vi "ControllerMain.vi"(0 "AllData":T1, 5 "PID gains":T5={"proportional gain (Kc)"=1.0, "integral time (Ti, min)"=0.01, "derivative time (Td, min)"=0.0} {"derivative time (Td, min)" format="%.3f"; "integral time (Ti, min)" format="%.3f"; "proportional gain (Kc)" format="%.3f"}, 7 "AdmittanceCoeffs":T4, 11 "error in (no error)":errorcluster) -> (4 "U1":dbl, 6 "Direction1":bool, 8 "U2":dbl, 10 "Direction 2":bool, 15 "error out":errorcluster)   [LabVIEW 2017, in "admittanceControllerLibrary.lvlib"]
doc: "The VI is the Admittance Controller Main API.\n\nInputs: All Data, PID Gains, Admittance Coeefficients.\n\nOutputs: Motor 1 demand and direction. Motor 2 demand and direction."
uses:
  admittanceControllerLibrary.lvlib
  Controls/AdmittanceGains.ctl
  TypeDefs/allData.ctl
  TypeDefs/dataOut.ctl
  TypeDefs/dataIn.ctl
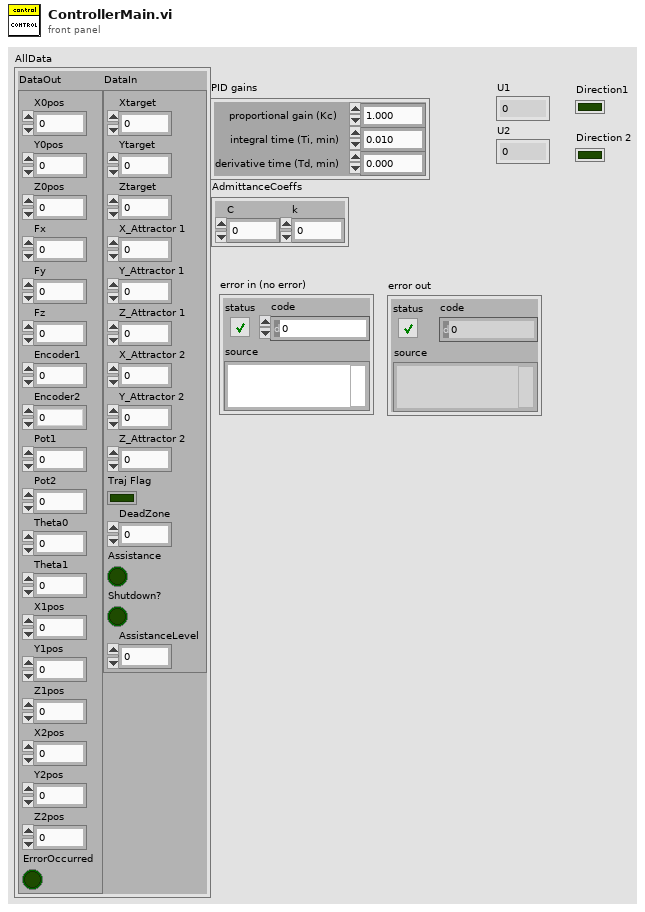
[diagram p1: front panel]
types:
  T1 = typedef "allData.ctl" = cluster{"DataOut":T2, "DataIn":T3}
  T2 = typedef "dataOut.ctl" = cluster{"X0pos":dbl, "Y0pos":dbl, "Z0pos":dbl, "Fx":dbl, "Fy":dbl, "Fz":dbl, "Encoder1":i32, "Encoder2":i32, "Pot1":dbl, "Pot2":dbl, "Theta0":dbl, "Theta1":dbl, "X1pos":dbl, "Y1pos":dbl, "Z1pos":dbl, "X2pos":dbl, "Y2pos":dbl, "Z2pos":dbl, "ErrorOccurred":bool}
  T3 = typedef "dataIn.ctl" = cluster{"Xtarget":dbl, "Ytarget":dbl, "Ztarget":dbl, "X_Attractor 1":dbl, "Y_Attractor 1":dbl, "Z_Attractor 1":dbl, "X_Attractor 2":dbl, "Y_Attractor 2":dbl, "Z_Attractor 2":dbl, "Traj Flag":bool, "DeadZone":dbl, "Assistance":bool, "Shutdown?":bool, "AssistanceLevel":dbl}
  T4 = typedef "admittanceControllerLibrary.lvlib/AdmittanceGains.ctl" = cluster{"C":dbl, "k":dbl}
  T5 = cluster{"proportional gain (Kc)":dbl, "integral time (Ti, min)":dbl, "derivative time (Td, min)":dbl}
  T6 = typedef "admittanceControllerLibrary.lvlib/ControlVariables.ctl" = cluster{"ControlFlag":bool, "Fx":dbl, "Fy":dbl, "Theta0":dbl, "Theta1":dbl, "CurrentX":dbl, "CurrentY":dbl, "TargetX":dbl, "TargetY":dbl, "DeadZone":dbl, "Assistance?":bool, "AssitanceLevel":dbl}
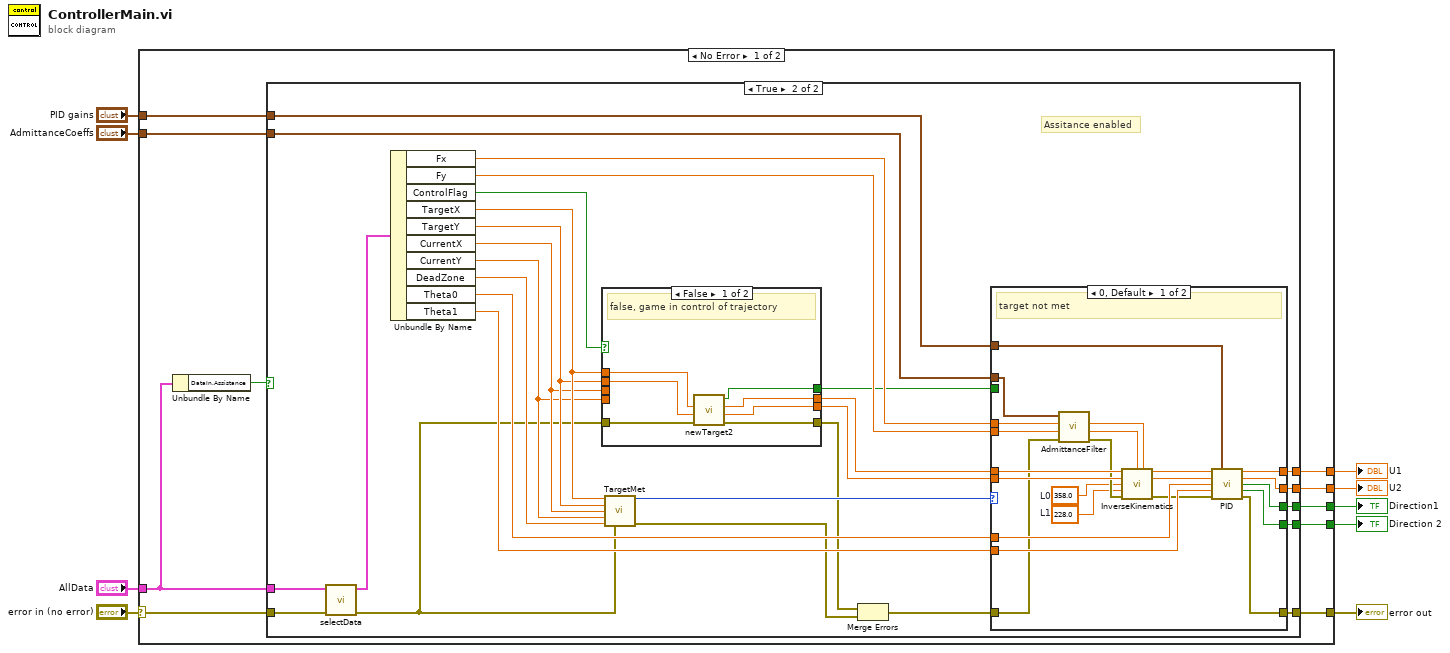
[diagram p0: block diagram]
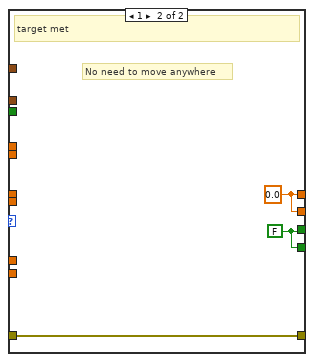
[diagram p3: hidden frame]
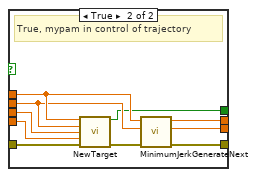
[diagram p4: hidden frame]
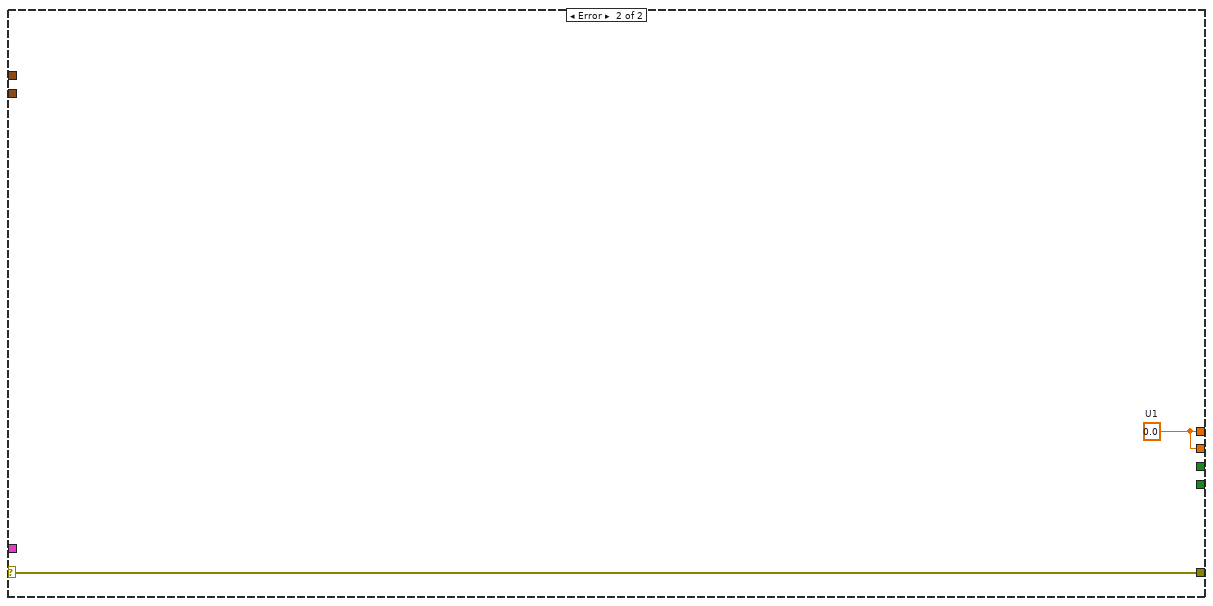
[diagram p5: hidden frame]
diagram:
  n1 = case shown="No Error" "error in (no error)" {
    selector: "error in (no error)" -> [w15 w92]
    tunnel: [w19 w91] -> w9
    tunnel: [w18 w91] -> w8
    tunnel: "PID gains" -> [w11 _]
    tunnel: "AdmittanceCoeffs" -> [w12 _]
    tunnel: [w17 _] -> w5
    tunnel: [w16 _] -> w4
    tunnel: [w14 w92] -> w2
    tunnel: "AllData" -> [w13 _]
    frame No Error {
      n2 = Unbundle By Name(w13) -> ("DataIn.Assistance"=w10:bool)
      n3 = case shown="True" w10 {
        tunnel: [_ w39] -> w19
        tunnel: [_ w38] -> w18
        tunnel: [_ w33] -> w17
        tunnel: [_ w32] -> w16
        tunnel: w15 -> [w20 w30]
        tunnel: [w20 w25] -> w14
        tunnel: w13 -> [_ w24]
        tunnel: w12 -> [_ w23]
        tunnel: w11 -> [_ w22]
        frame False {
          # "Assistance not enabled"
        }
        frame True {
          # "Assitance enabled"
          n4 = call "selectData.vi"("error in (no error)"=w30, "AllData"=w24) -> ("error out"=w27:errorcluster, 3:w31:T6)  [unwired: 8 in]
          n5 = Unbundle By Name(w31) -> ("Fx"=w36:dbl, "Fy"=w37:dbl, "ControlFlag"=w48:bool, "TargetX"=w47:dbl, "TargetY"=w46:dbl, "CurrentX"=w45:dbl, "CurrentY"=w44:dbl, "DeadZone"=w43:dbl, "Theta0"=w34:dbl, "Theta1"=w35:dbl)
          n6 = case shown="False" w48 {
            tunnel: w47 -> [w75 w88]
            tunnel: w46 -> [w74 w87]
            tunnel: w45 -> [_ w86]
            tunnel: w44 -> [_ w85]
            tunnel: [w77 w90] -> w41
            tunnel: [w78 w89] -> w40
            tunnel: w27 -> [w80 w84]
            tunnel: [w79 w82] -> w29
            tunnel: [w76 w81] -> w21
            frame False {
              # "false, game in control of trajectory"
              n7 = call "newTarget2.vi"("error in (no error)"=w80, "Target Y"=w74, "Target X"=w75) -> ("error out"=w79:errorcluster, "Target y"=w78:dbl, "Target x"=w77:dbl, "NewTarget"=w76:bool)  [unwired: 5 in]
            }
            frame True {
              # "True, mypam in control of trajectory"
              n8 = call "NewTarget.vi"("Target x"=w88, "Target y"=w87, "Current x"=w86, "Current y"=w85, "error in (no error)"=w84) -> ("NewTarget"=w81:bool, "error out"=w83:errorcluster)  [unwired: 9 in]
              n9 = call "MinimumJerkGenerateNext.vi"("error in (no error)"=w83, "Target y"=w87, "Target x"=w88) -> ("error out"=w82:errorcluster, "yt"=w89:dbl, "xt"=w90:dbl)  [unwired: 6 in]
            }
          }
          n10 = call "TargetMet.vi"("Target x (mm)"=w47, "Target y (mm)"=w46, "Current x (mm)"=w45, "Current y (mm)"=w44, "Dead Zone (mm)"=w43, "error in (no error)"=w27) -> ("out"=w42:i32, "error out"=w28:errorcluster)  [unwired: 8 in]
          n11 = Merge Errors(w29, w28) -> (w26:errorcluster)
          n12 = case shown="0, Default" w42 {
            tunnel: w41 -> [w61 _]
            tunnel: w40 -> [w60 _]
            tunnel: [w66 w73] -> w39
            tunnel: [w67 w73] -> w38
            tunnel: w36 -> [w63 _]
            tunnel: w37 -> [w62 _]
            tunnel: w34 -> [w69 _]
            tunnel: w35 -> [w68 _]
            tunnel: w22 -> [w70 _]
            tunnel: [w65 w72] -> w33
            tunnel: [w64 w72] -> w32
            tunnel: w26 -> [w56 w71]
            tunnel: [w58 w71] -> w25
            tunnel: w23 -> [w49 _]
            tunnel: w21 -> [_ _]
            frame 0, Default {
              w50 = 228.0  # L1
              w51 = 358.0  # L0
              # "target not met"
              n13 = call "AdmittanceFilter.vi"("error in (no error)"=w56, "Fy"=w62, "Fx"=w63, "AdmittanceCoeffs"=w49) -> ("error out"=w57:errorcluster, "Delta y"=w55:dbl, "Delta x"=w54:dbl)  [unwired: 5 in]
              n14 = call "InverseKinematics.vi"("Next X"=w61, "deltaY"=w55, "deltaX"=w54, "Next Y"=w60, "L0"=w51, "L1"=w50, "error in (no error)"=w57) -> ("destheta0"=w53:dbl, "destheta1"=w52:dbl, "error out"=w59:errorcluster)  [unwired: 6 in]
              n15 = call "PID.vi"("Des theta0"=w53, "PID gains"=w70, "Des theta1"=w52, "current theta0"=w69, "current theta1"=w68, "error in (no error)"=w59) -> ("U1"=w67:dbl, "U2"=w66:dbl, "Dir1"=w65:bool, "Dir2"=w64:bool, "error out"=w58:errorcluster)  [unwired: 5 in]
            }
            frame 1 {
              w72 = FALSE
              w73 = 0.0 ("U1")
              # "No need to move anywhere"
              # "target met"
            }
          }
        }
      }
    }
    frame Error {
      w91 = 0.0  # U1
    }
  }
  "U1" <- w8
  "U2" <- w9
  "Direction1" <- w5
  "Direction 2" <- w4
  "error out" <- w2
